vi "Gain.vi"(0 "stream in":T1, 1 "gain":dbl) -> (2 "stream out":T1)   [LabVIEW 2023]
uses:
  <extravilib>/ChannelInstances/Stream-dbl/)Channel.ctl
  <extravilib>/ChannelInstances/Stream-dbl/Read With Abort.vi
  <extravilib>/ChannelInstances/Stream-dbl/Write With Abort.vi
  <extravilib>/ChannelInstances/Stream-dbl/EndpointRead.vi
  <extravilib>/ChannelInstances/Stream-dbl/Endpoint.vi
  <extravilib>/ChannelInstances/Stream-dbl/)Channel.vi
  <resource>/ChannelSupport/_ChannelSupport/WaitIfNeeded.vi
  <extravilib>/ChannelInstances/Stream-dbl.lvlib
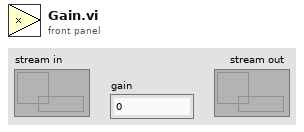
[diagram p1: front panel]
types:
  T1 = typedef "Stream-dbl.lvlib/)Channel.ctl" = refnum<queue>
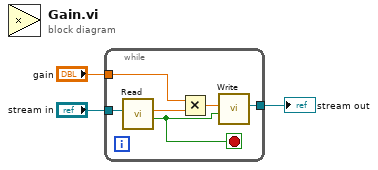
[diagram p0: block diagram]
diagram:
  n1 = while {
    tunnel: [w5] -> w2
    tunnel: "stream in" -> [w8]
    tunnel: "gain" -> [w9]
    stop <- w4 stop-if-true
    n2 = call <extravilib>:"Read.vi"("channel"=w8) -> ("last element?"=w4:bool, "element"=w7:dbl)  [unwired: 6 in, 3 out]
    n3 = Multiply(x=w9, y=w7) -> (x*y=w6:dbl)
    n4 = call <extravilib>:"Write.vi"("last element? (F)"=w4, "element"=w6) -> ("channel"=w5:T1)  [unwired: 7 in, 2 out]
  }
  "stream out" <- w2
